vi "Detect Construction Zone.vi"(11 "Task coordinate (cm)":dbl[](array[numeric])) -> (3 "In construction zone?":bool)   [LabVIEW 2017]
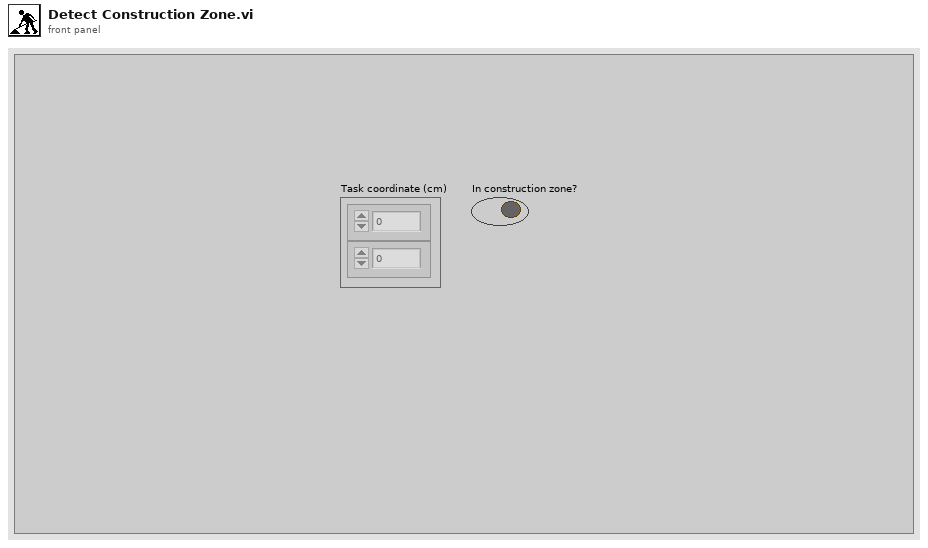
[diagram p1: front panel]
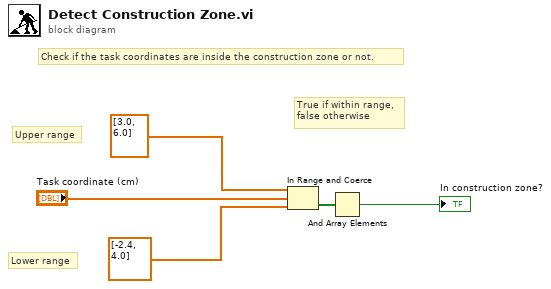
[diagram p0: block diagram]
diagram:
  # "Check if the task coordinates are inside the construction zone or not."
  # "True if within range,\nfalse otherwise"
  # "Lower range"
  # "Upper range"
  n1 = In Range and Coerce(upper limit=dbl[] [3.0, 6.0], x="Task coordinate (cm)", lower limit=dbl[] [-2.4, 4.0]) -> (In Range?=w4:bool[])  [unwired: 1 out]
  n2 = And Array Elements(Boolean array=w4) -> (logical AND=→"In construction zone?":bool)
